vi "Run Tests - When Tests Provided - Executes Test.vi"() -> ()   [LabVIEW 2017, in "LVUnit Test Executor.Tests.lvlib"]
uses:
  LVUnit Test Executor.Tests.lvlib
  LVUnit Test Executor/LVUnit Test Executor.lvclass
  LVUnit Test Case/LVUnit Test Case.lvclass
  C:/Users/pasca/source/repos/lvunit/Test Case/Test Case.lvclass
  Assertion/Assertion.lvlib
  Test Case/Test Case.lvclass
panel:
  out "error out":errorcluster
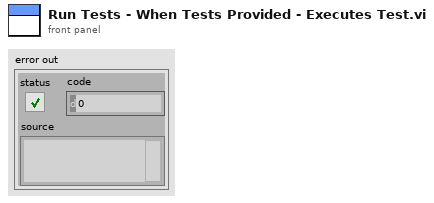
[diagram p1: front panel]
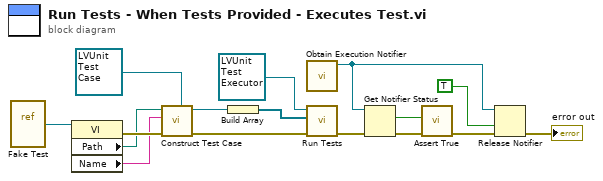
[diagram p0: block diagram]
diagram:
  n1 = vi-ref "Fake Test.vi"() -> (w8:refnum<vi>)
  n2 = property class="VI"(reference=w8) -> (error out=w7:errorcluster, "Path"=w6:path, "Name"=w5:string)  [unwired: 1 in, 1 out]
  n3 = call "Construct Test Case.vi"("Test Case in"=refnum<class "LVUnit Test Case.lvclass"> refnum ("LVUnit Test Case"), "error in (no error)"=w7, "Qualified Name"=w5, "Path"=w6) -> ("error out"=w4:errorcluster, "Test Case out"=w3:refnum<class "LVUnit Test Case.lvclass">)  [unwired: 6 in]
  n4 = Build Array(w3) -> (w2:refnum<class "LVUnit Test Case.lvclass">[])
  n5 = call "Obtain Execution Notifier.vi"() -> ("Execution Notifier"=w11:refnum<notifier>)  [unwired: 11 in]
  n6 = call-dynamic "Run Tests.vi"("error in (no error)"=w4, "Test Cases"=w2, "LVUnit Test Executor in"=refnum<class "LVUnit Test Executor.lvclass"> refnum ("LVUnit Test Executor")) -> ("error out"=w15:errorcluster)  [unwired: 6 in, 2 out]
  n7 = Get Notifier Status(notifier=w11, error in (no error)=w15) -> (current notification=w14:bool, error out=w9:errorcluster)  [unwired: 3 out]
  n8 = call "Assert True.vi"("error in (no error)"=w9, "Condition"=w14) -> ("error out"=w13:errorcluster)  [unwired: 9 in]
  n9 = Release Notifier(notifier=w11, force destroy? (F)=TRUE, error in (no error)=w13) -> (error out=→"error out":errorcluster)  [unwired: 2 out]
